vi "NB_ReadProperty.vi"(8 "Error In":errorcluster, 11 "object in":refnum<class "NativeBaseTemplate_4x4x4.lvclass">) -> (0 "Error Out":errorcluster, 2 "property":bool, 3 "object out":refnum<class "NativeBaseTemplate_4x4x4.lvclass">)   [LabVIEW 2020, in "NativeBaseTemplate_4x4x4.lvclass"]
uses:
  NativeBaseTemplate_4x4x4.lvclass
  NativeBaseTemplate_4x4x4.lvclass/NativeBaseTemplate_4x4x4.ctl
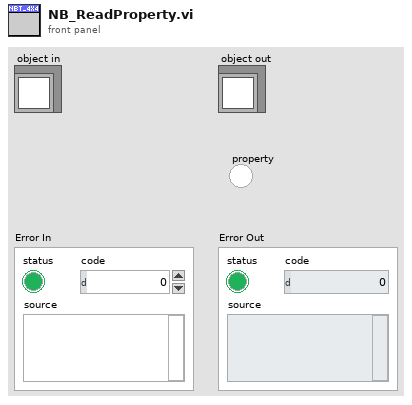
[diagram p1: front panel]
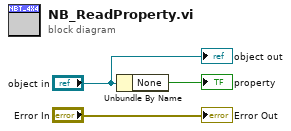
[diagram p0: block diagram]
diagram:
  n1 = Unbundle By Name("object in") -> ("None"=→"property":bool)
  "Error Out" <- "Error In"
  "object out" <- "object in"
